vi "FTW-CodeGen-Callback-FindGObject.vi"(4 "context in":variant, 5 "objref":refnum<vi>) -> (1 "context out":variant, 2 "traverse flags":i32 format="0x%08x")   [LabVIEW 2015]
panel:
  # "Inputs"
  # "Outputs"
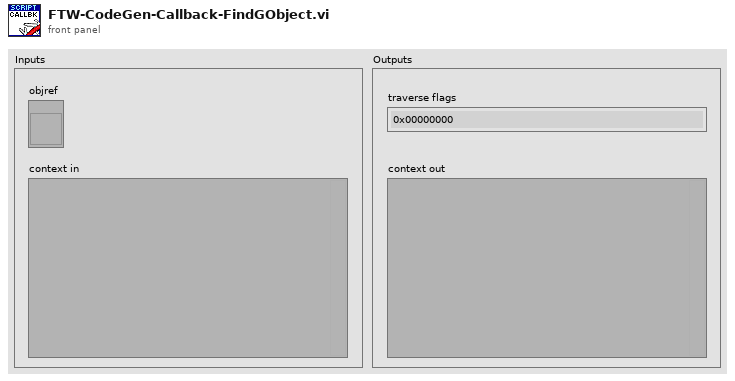
[diagram p1: front panel]
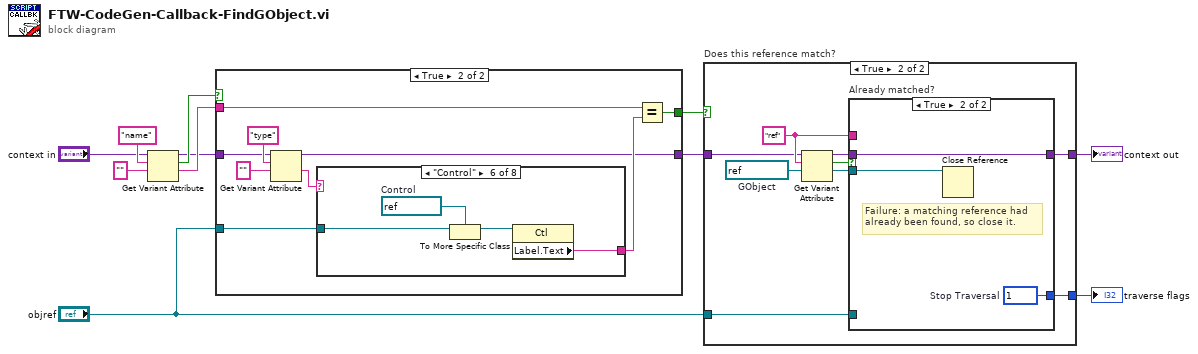
[diagram p0: block diagram]
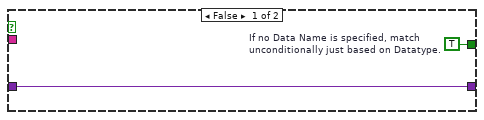
[diagram p2: hidden frame]
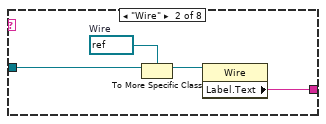
[diagram p4: hidden frame]
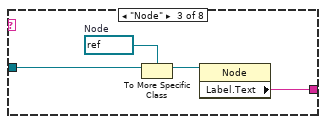
[diagram p5: hidden frame]
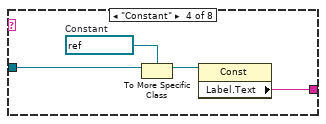
[diagram p6: hidden frame]
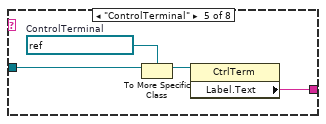
[diagram p7: hidden frame]
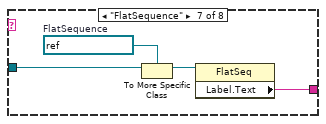
[diagram p8: hidden frame]
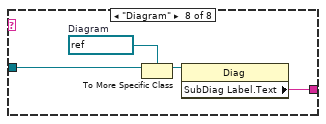
[diagram p9: hidden frame]
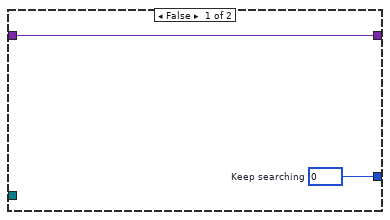
[diagram p10: hidden frame]
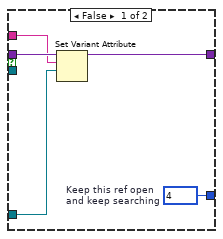
[diagram p11: hidden frame]
diagram:
  n1 = Get Variant Attribute(Variant="context in", name="name", default value (empty Variant)="") -> (duplicate Variant=w2:variant, found=w6:bool, value=w7:string)  [unwired: 1 in, 1 out]
  n2 = case shown="True" w6 {
    tunnel: "objref" -> [_ w17]
    tunnel: w7 -> [_ w22]
    tunnel: [w13 w16] -> w5
    tunnel: w2 -> [w12 w19]
    tunnel: [w12 w14] -> w1
    frame False {
      w13 = TRUE  # If no Data Name is specified, match unconditionally just based on Datatype.
    }
    frame True {
      n3 = Get Variant Attribute(Variant=w19, name="type", default value (empty Variant)="") -> (duplicate Variant=w14:variant, value=w18:string)  [unwired: 1 in, 2 out]
      n4 = case shown="\"Control\"" w18 {
        tunnel: w17 -> [_ w25 w29 w33 w37 w41 w45 w49]
        tunnel: [_ w23 w27 w31 w35 w39 w43 w47] -> w15
        frame Default {
          # "This is not a class type\nknown to have a label."
        }
        frame "Wire" {
          w26 = refnum<vi> refnum  # Wire
          n5 = To More Specific Class(target class=w26, reference=w25) -> (specific class reference=w24:refnum<vi>)  [unwired: 1 in, 1 out]
          n6 = property class="Wire"(reference=w24) -> ("Label.Text"=w23:string)  [unwired: 1 in, 2 out]
        }
        frame "Node" {
          w30 = refnum<vi> refnum  # Node
          n7 = To More Specific Class(target class=w30, reference=w29) -> (specific class reference=w28:refnum<vi>)  [unwired: 1 in, 1 out]
          n8 = property class="Node"(reference=w28) -> ("Label.Text"=w27:string)  [unwired: 1 in, 2 out]
        }
        frame "Constant" {
          w34 = refnum<vi> refnum  # Constant
          n9 = To More Specific Class(target class=w34, reference=w33) -> (specific class reference=w32:refnum<vi>)  [unwired: 1 in, 1 out]
          n10 = property class="Const"(reference=w32) -> ("Label.Text"=w31:string)  [unwired: 1 in, 2 out]
        }
        frame "ControlTerminal" {
          w38 = refnum<vi> refnum  # ControlTerminal
          n11 = To More Specific Class(target class=w38, reference=w37) -> (specific class reference=w36:refnum<vi>)  [unwired: 1 in, 1 out]
          n12 = property class="CtrlTerm"(reference=w36) -> ("Label.Text"=w35:string)  [unwired: 1 in, 2 out]
        }
        frame "Control" {
          w42 = refnum<vi> refnum  # Control
          n13 = To More Specific Class(target class=w42, reference=w41) -> (specific class reference=w40:refnum<vi>)  [unwired: 1 in, 1 out]
          n14 = property class="Ctl"(reference=w40) -> ("Label.Text"=w39:string)  [unwired: 1 in, 2 out]
        }
        frame "FlatSequence" {
          w46 = refnum<vi> refnum  # FlatSequence
          n15 = To More Specific Class(target class=w46, reference=w45) -> (specific class reference=w44:refnum<vi>)  [unwired: 1 in, 1 out]
          n16 = property class="FlatSeq"(reference=w44) -> ("Label.Text"=w43:string)  [unwired: 1 in, 2 out]
        }
        frame "Diagram" {
          w50 = refnum<vi> refnum  # Diagram
          n17 = To More Specific Class(target class=w50, reference=w49) -> (specific class reference=w48:refnum<vi>)  [unwired: 1 in, 1 out]
          n18 = property class="Diag"(reference=w48) -> ("SubDiag Label.Text"=w47:string)  [unwired: 1 in, 2 out]
        }
      }
      n19 = Equal?(x=w22, y=w15) -> (x = y?=w16:bool)
    }
  }
  n20 = case "Does this reference match?" shown="True" w5 {
    tunnel: [w52 w61] -> w11
    tunnel: "objref" -> [_ w60]
    tunnel: w1 -> [w52 w55]
    tunnel: [w51 w59] -> w4
    frame False {
      w51 = 0  # Keep searching
    }
    frame True {
      w58 = refnum<vi> refnum  # GObject
      w57 = "ref" ("name")
      n21 = Get Variant Attribute(Variant=w55, name=w57, default value (empty Variant)=w58) -> (duplicate Variant=w56:variant, found=w54:bool, value=w53:refnum<vi>)  [unwired: 1 in, 1 out]
      n22 = case "Already matched?" shown="True" w54 {
        tunnel: w57 -> [w63 _]
        tunnel: [w65 w68] -> w61
        tunnel: w53 -> [_ w67]
        tunnel: w60 -> [w62 _]
        tunnel: w56 -> [w66 w68]
        tunnel: [w64 w69] -> w59
        frame False {
          w64 = 4  # Keep this ref open and keep searching
          n23 = Set Variant Attribute(Variant=w66, name=w63, value=w62) -> (Variant out=w65:variant)  [unwired: 1 in, 2 out]
        }
        frame True {
          w69 = 1  # Stop Traversal
          # "Failure: a matching reference had\nalready been found, so close it."
          n24 = Close Reference(reference=w67) -> ()  [unwired: 1 in, 1 out]
        }
      }
    }
  }
  "traverse flags" <- w4
  "context out" <- w11
